vi "Retrive Data.vi"(8 "error in (no error)":errorcluster, 9 "Tag":string, 10 "Tree In":refnum<class "Tree.lvclass">, 11 "Tree Data Folder in":refnum<class "Tree Data Folder.lvclass">) -> (0 "error out":errorcluster, 1 "Data Out":T1, 2 "Tree Out":refnum<class "Tree.lvclass">, 3 "Tree Data Folder out":refnum<class "Tree Data Folder.lvclass">, 5 "Data Group Out":T1[](array[typedef]))   [LabVIEW 2024, in "Tree Data Folder.lvclass"]
uses:
  Tree Data Folder.lvclass
  Tree/Tree.lvclass
  Tree/Type Def/Tree Item.ctl
  Tree Data Folder.lvclass/Tree Data Folder.ctl
  Composite Tree Data/Composite Tree Data.lvclass
  Tree Data File/Tree Data File.lvclass
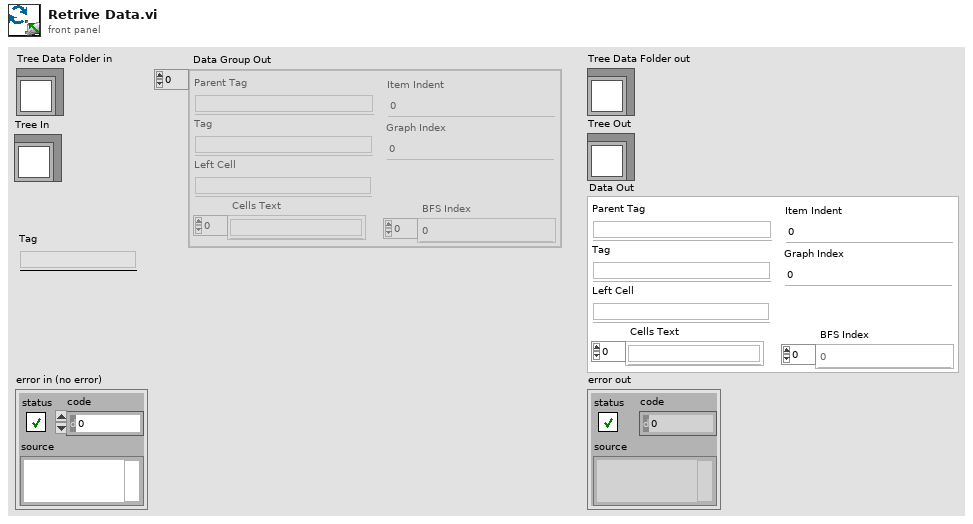
[diagram p1: front panel]
types:
  T1 = typedef "Tree Item.ctl" = cluster{"Parent Tag":string, "Tag":string, "Left Cell":string, "Cells Text":string[], "BFS Index":i32[], "Graph Index":i32, "Item Indent":i32}
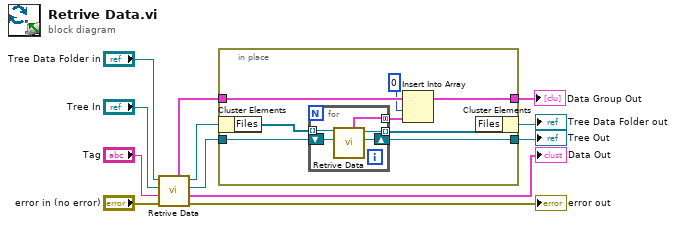
[diagram p0: block diagram]
diagram:
  n1 = call-parent "Retrive Data.vi"("error in (no error)"="error in (no error)", "Tag"="Tag", "Tree In"="Tree In", "Composite Tree Data in"="Tree Data Folder in") -> ("error out"=→"error out":errorcluster, "Data Out"=→"Data Out":T1, "Tree Out"=w6:refnum<class "Tree.lvclass">, "Composite Tree Data out"=w5:refnum<class "Tree Data Folder.lvclass">, "Data Group Out"=w4:T1[])  [unwired: 3 in]
  n2 = in-place {
    in-place-border: w4 -> [w16]
    in-place-border: w6 -> [w18]
    in-place-border: [w17] -> w3
    in-place-border: [w13] -> w1
    n3 = in-place-cluster #1(w5) -> ("Files"=w20:refnum<class "Tree Data File.lvclass">[])
    n4 = for {
      tunnel: w20 -> [w25] mode=indexing
      tunnel: [w24] -> w19 mode=indexing
      shift-right: [w22] -> w17
      shift-left: w18 -> [w23]
      tunnel: [w21] -> w15 mode=concatenating
      n5 = call-dynamic "Retrive Data.vi"("Tree In"=w23, "Composite Tree Data in"=w25) -> ("Tree Out"=w22:refnum<class "Tree.lvclass">, "Composite Tree Data out"=w24:refnum<class "Tree Data File.lvclass">, "Data Group Out"=w21:T1[])  [unwired: 5 in, 2 out]
    }
    n6 = Insert Into Array(array=w16, index=0, new element=w15) -> (w13:T1[])
    n7 = in-place-cluster #1("Files"=w19) -> (→"Tree Data Folder out":refnum<class "Tree Data Folder.lvclass">)
  }
  "Tree Out" <- w3
  "Data Group Out" <- w1
